vi "TestJ1.vi"() -> ()   [LabVIEW 2009]
panel:
  out "output cluster":T1
  in  "file path (use dialog)":path
  out "Data Out":i32[](array[numeric])
  in  "FPGA IP Address":string
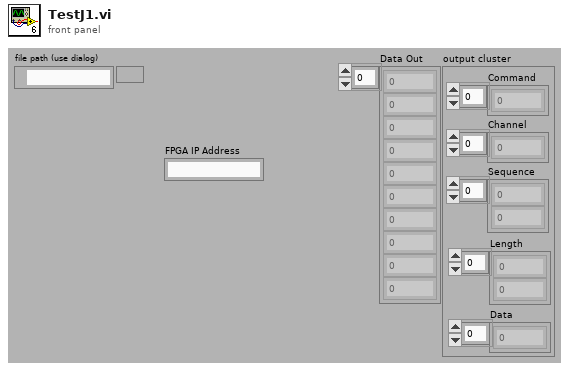
[diagram p1: front panel]
types:
  T1 = cluster{"Command":i32[], "Channel":i32[], "Sequence":i32[], "Length":i32[], "Data":i32[]}
  T2 = enum16{"open", "replace", "create", "open or create", "replace or create", "replace or create with confirmation"}
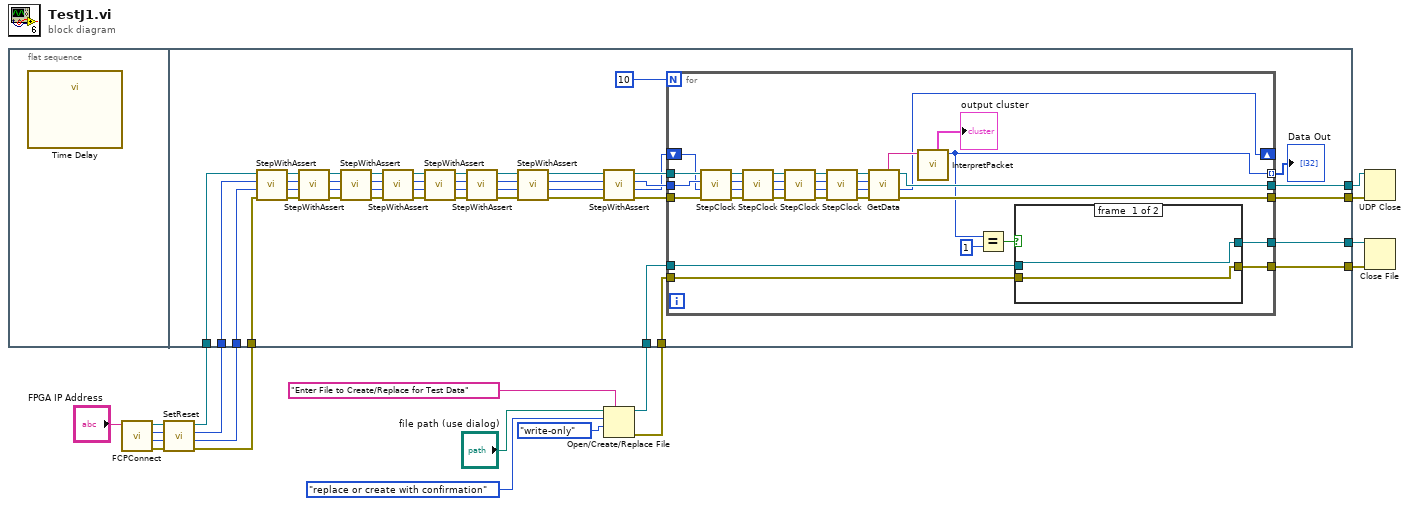
[diagram p0: block diagram]
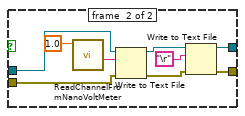
[diagram p2: hidden frame]
diagram:
  n1 = flat-sequence {
    tunnel: w14 -> [w51]
    tunnel: w13 -> [w50]
    tunnel: w12 -> [w49]
    tunnel: w11 -> [w48]
    tunnel: [w59] -> w10
    tunnel: [w58] -> w9
    tunnel: w4 -> [w55]
    tunnel: w3 -> [w54]
    tunnel: [w53] -> w2
    tunnel: [w52] -> w1
    frame #0 {
      n2 = call "Time Delay"() -> ()  [unwired: 11 in, 1 out]
    }
    frame #1 {
      n3 = call "StepWithAssert.vi"("error in (no error)"=w48, "SequenceNumber"=w49, "address"=w50, "connection ID"=w51) -> ("error out"=w40:errorcluster, "SequenceNumber out"=w41:i32, "address out"=w42:u32, "connection ID out"=w43:refnum<k16>)  [unwired: 4 in]
      n4 = call "StepWithAssert.vi"("error in (no error)"=w40, "SequenceNumber"=w41, "address"=w42, "connection ID"=w43) -> ("error out"=w44:errorcluster, "SequenceNumber out"=w45:i32, "address out"=w46:u32, "connection ID out"=w47:refnum<k16>)  [unwired: 4 in]
      n5 = call "StepWithAssert.vi"("error in (no error)"=w44, "SequenceNumber"=w45, "address"=w46, "connection ID"=w47) -> ("error out"=w36:errorcluster, "SequenceNumber out"=w37:i32, "address out"=w38:u32, "connection ID out"=w39:refnum<k16>)  [unwired: 4 in]
      n6 = call "StepWithAssert.vi"("error in (no error)"=w36, "SequenceNumber"=w37, "address"=w38, "connection ID"=w39) -> ("error out"=w35:errorcluster, "SequenceNumber out"=w34:i32, "address out"=w33:u32, "connection ID out"=w32:refnum<k16>)  [unwired: 4 in]
      n7 = call "StepWithAssert.vi"("error in (no error)"=w35, "SequenceNumber"=w34, "address"=w33, "connection ID"=w32) -> ("error out"=w31:errorcluster, "SequenceNumber out"=w30:i32, "address out"=w29:u32, "connection ID out"=w28:refnum<k16>)  [unwired: 4 in]
      n8 = call "StepWithAssert.vi"("error in (no error)"=w31, "SequenceNumber"=w30, "address"=w29, "connection ID"=w28) -> ("error out"=w27:errorcluster, "SequenceNumber out"=w26:i32, "address out"=w25:u32, "connection ID out"=w24:refnum<k16>)  [unwired: 4 in]
      n9 = call "StepWithAssert.vi"("error in (no error)"=w27, "SequenceNumber"=w26, "address"=w25, "connection ID"=w24) -> ("error out"=w23:errorcluster, "SequenceNumber out"=w22:i32, "address out"=w21:u32, "connection ID out"=w20:refnum<k16>)  [unwired: 4 in]
      n10 = call "StepWithAssert.vi"("error in (no error)"=w23, "SequenceNumber"=w22, "address"=w21, "connection ID"=w20) -> ("error out"=w60:errorcluster, "SequenceNumber out"=w56:i32, "address out"=w61:u32, "connection ID out"=w62:refnum<k16>)  [unwired: 4 in]
      n11 = for {
        N: 10 -> [_]
        tunnel: w62 -> [w94]
        tunnel: w61 -> [w93]
        tunnel: w60 -> [w92]
        tunnel: [w91] -> w59
        tunnel: [w90] -> w58
        tunnel: [w84] -> w57 mode=indexing
        shift-right: [w89] -> _
        shift-left: w56 -> [w88]
        tunnel: w55 -> [w86]
        tunnel: w54 -> [w85]
        tunnel: [w82] -> w53
        tunnel: [w81] -> w52
        n12 = call "StepClock.vi"("error in (no error)"=w92, "SequenceNumber"=w88, "address"=w93, "connection ID"=w94) -> ("error out"=w77:errorcluster, "SequenceNumber out"=w78:i32, "address out"=w79:u32, "connection ID out"=w80:refnum<k16>)  [unwired: 4 in]
        n13 = call "StepClock.vi"("error in (no error)"=w77, "SequenceNumber"=w78, "address"=w79, "connection ID"=w80) -> ("error out"=w76:errorcluster, "SequenceNumber out"=w75:i32, "address out"=w74:u32, "connection ID out"=w73:refnum<k16>)  [unwired: 4 in]
        n14 = call "StepClock.vi"("error in (no error)"=w76, "SequenceNumber"=w75, "address"=w74, "connection ID"=w73) -> ("error out"=w69:errorcluster, "SequenceNumber out"=w70:i32, "address out"=w71:u32, "connection ID out"=w72:refnum<k16>)  [unwired: 4 in]
        n15 = call "StepClock.vi"("error in (no error)"=w69, "SequenceNumber"=w70, "address"=w71, "connection ID"=w72) -> ("error out"=w65:errorcluster, "SequenceNumber out"=w66:i32, "address out"=w67:u32, "connection ID out"=w68:refnum<k16>)  [unwired: 4 in]
        n16 = call "GetData.vi"("error in (no error)"=w65, "SequenceNumber"=w66, "address"=w67, "connection ID"=w68) -> ("error out"=w90:errorcluster, "SequenceNumber out"=w89:i32, "connection ID out"=w91:refnum<k16>, "data out"=w95:string)  [unwired: 3 in, 1 out]
        n17 = call "InterpretPacket.vi"("Data In"=w95) -> ("Data Out"=w84:u8, "output cluster"=→"output cluster":T1)  [unwired: 9 in]
        n18 = Equal?(x=w84, y=u8 1) -> (x = y?=w87:bool)
        n19 = case shown="True" w87 {
          tunnel: w86 -> [w97 w106]
          tunnel: w85 -> [w96 w105]
          tunnel: [w97 w101] -> w82
          tunnel: [w96 w100] -> w81
          frame #0 {
          }
          frame #1 {
            n20 = call "ReadChannelFromNanoVoltMeter.vi"("ChannelSelection"=1.0) -> ("String Measurement"=w98:string)  [unwired: 8 in, 2 out]
            n21 = Write to Text File(file (use dialog)=w106, text=w98, error in=w105) -> (refnum out=w104:refnum<file>, error out=w103:errorcluster)  [unwired: 1 in, 1 out]
            n22 = Write to Text File(file (use dialog)=w104, text="\r", error in=w103) -> (refnum out=w101:refnum<file>, error out=w100:errorcluster)  [unwired: 1 in, 1 out]
          }
        }
      }
      "Data Out" <- w57
    }
  }
  n23 = call "FCPConnect.vi"("FPGA IP Address"="FPGA IP Address") -> ("error out"=w17:errorcluster, "Sequence Number"=w15:i32, "FPGA IP Address Out"=w16:u32, "connection ID out"=w18:refnum<k16>)  [unwired: 7 in]
  n24 = call "SetReset.vi"("error in (no error)"=w17, "SequenceNumber"=w15, "address"=w16, "connection ID"=w18) -> ("error out"=w11:errorcluster, "SequenceNumber out"=w12:i32, "Address out"=w13:u32, "connection ID out"=w14:refnum<k16>)  [unwired: 4 in]
  n25 = Open/Create/Replace File(file path (use dialog)="file path (use dialog)", prompt="Enter File to Create/Replace for Test Data", operation (0:open)=T2."replace or create with confirmation", access (0:read/write)=enum16{"read/write", "read-only", "write-only"}."write-only") -> (refnum out=w4:refnum<file>, error out=w3:errorcluster)  [unwired: 2 in, 1 out]
  n26 = UDP Close(connection ID=w10, 8:w9) -> ()  [unwired: 2 out]
  n27 = Close File(refnum=w2, error in=w1) -> ()  [unwired: 2 out]
